vi "CTRE_Phoenix_CANcoder_SetPositionPolymorphic.vi"   [LabVIEW 2019]
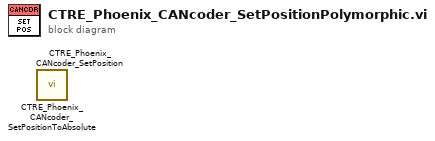
[diagram p0: block diagram]
diagram:
  n1 = call <vilib>:"CTRE_Phoenix_CANcoder_SetPositionToAbsolute.vi"() -> ()  [unwired: 10 in, 2 out]
  n2 = call <vilib>:"CTRE_Phoenix_CANcoder_SetPosition.vi"() -> ()  [unwired: 10 in, 2 out]
